vi "Filter Number.vi"(7 "Filter Number":i32, 8 "error in (no error)":errorcluster, 11 "VISA resource name":refnum<visa-resource-name>) -> (0 "error out":errorcluster, 2 "Connected? 2":bool, 3 "VISA resource name out":refnum<visa-resource-name>)   [LabVIEW 2018]
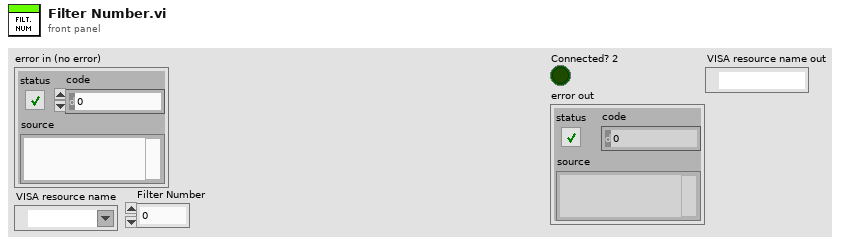
[diagram p1: front panel]
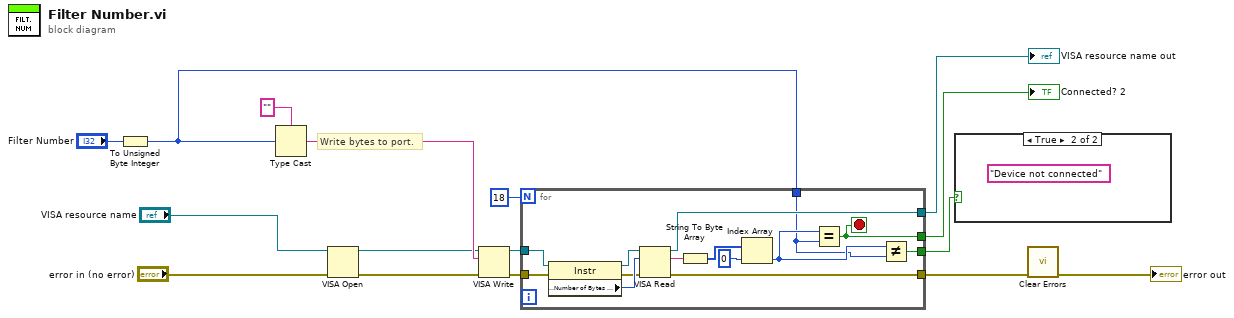
[diagram p0: block diagram]
diagram:
  # "Write bytes to port."
  n1 = To Unsigned Byte Integer(number="Filter Number") -> (unsigned 8bit integer=w1:u8)
  n2 = Type Cast(type="", x=w1) -> (*(type *) &x=w12:string)
  n3 = VISA Open(error in (no error)="error in (no error)", VISA resource name="VISA resource name") -> (VISA resource name=w11:refnum<visa-resource-name>, error out=w10:errorcluster)  [unwired: 3 in]
  n4 = VISA Write(VISA resource name=w11, write buffer=w12, error in (no error)=w10) -> (VISA resource name out=w13:refnum<visa-resource-name>, error out=w14:errorcluster)  [unwired: 1 out]
  n5 = for {
    N: 18 -> [_]
    tunnel: w13 -> [w24]
    tunnel: w14 -> [w25]
    tunnel: [w27] -> w4
    tunnel: [w26] -> w5
    tunnel: [w20] -> w15
    tunnel: [w18] -> w16
    tunnel: w1 -> [w17]
    stop <- w20 stop-if-true
    n6 = property class="Instr"(reference=w24, error in=w25) -> (reference out=w23:refnum<visa-resource-name>, error out=w21:errorcluster, "Serial Settings:Number of Bytes at Serial Port"=w22:u32)
    n7 = VISA Read(VISA resource name=w23, byte count=w22, error in (no error)=w21) -> (VISA resource name out=w27:refnum<visa-resource-name>, read buffer=w30:string, error out=w26:errorcluster)  [unwired: 1 out]
    n8 = String To Byte Array(string=w30) -> (unsigned byte array=w29:u8[])
    n9 = Index Array(array=w29, index=0) -> (element=w19:u8)
    n10 = Equal?(x=w19, y=w17) -> (x = y?=w20:bool)
    n11 = Not Equal?(x=w19, y=w17) -> (x != y?=w18:bool)
  }
  "Connected? 2" <- w15
  "VISA resource name out" <- w4
  n12 = case shown="True" w16 {
    frame False {
    }
    frame True {
      (unwired) "Device not connected"
    }
  }
  n13 = call <vilib>:"Clear Errors.vi"("error in (no error)"=w5) -> ("error out"=→"error out":errorcluster)  [unwired: 5 in, 1 out]
